vi "RWRPrompt.vi"(0 "Value Present in Detector 2":string) -> (1 "Value to update in Detector 2":string="0000", 2 "Cancel Pressed":bool)   [LabVIEW 2018]
panel:
  in  "Cancel":bool
  in  "Update":bool
  in  "Value to update in Detector":string="0000"
  out "Value Present in Detector":string
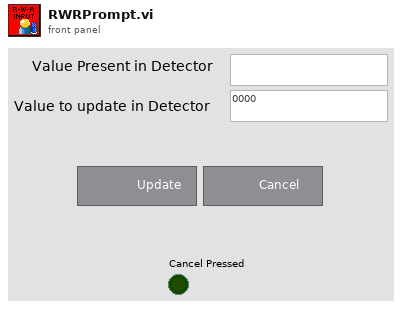
[diagram p1: front panel]
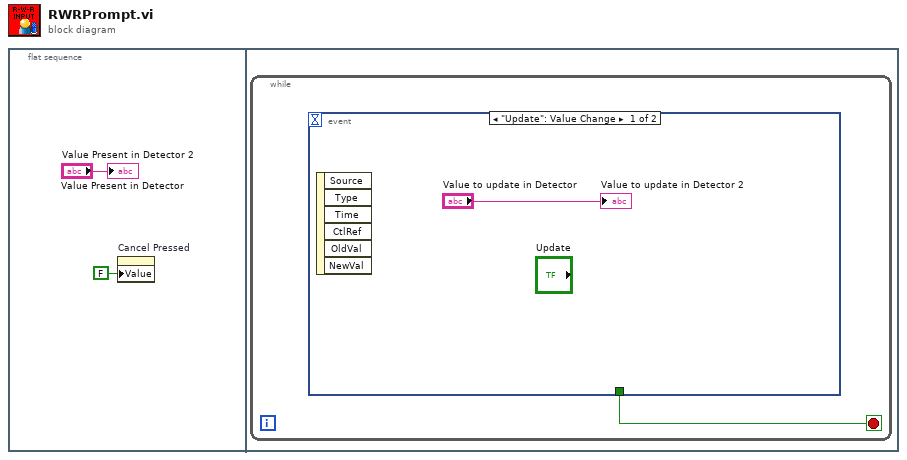
[diagram p0: block diagram]
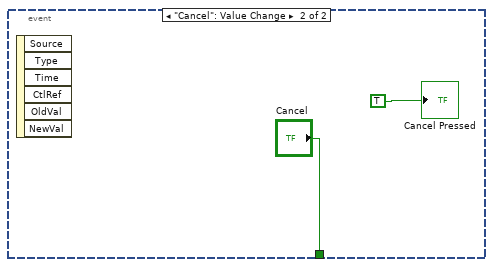
[diagram p2: hidden frame]
diagram:
  n1 = flat-sequence {
    frame #0 {
      n2 = property on="Cancel Pressed" class="Bool (strict)"("Value"=FALSE ("Cancel Pressed")) -> ()  [unwired: 2 in, 2 out]
      "Value Present in Detector" <- "Value Present in Detector 2"
    }
    frame #1 {
      n3 = while {
        stop <- w3 stop-if-true
        n4 = event shown="[0] \"Update\": Value Change" {
          selector: _ -> [_ _]
          dyn-events: _ -> [_ _]
          timeout: _ -> [_ _]
          tunnel: [_ "Cancel"] -> w3
          event "Update": Value Change {
            n5 = event-data() -> ()  [unwired: 1 in, 6 out]
            "Value to update in Detector 2" <- "Value to update in Detector"
          }
          event "Cancel": Value Change {
            n6 = event-data() -> ()  [unwired: 1 in, 6 out]
            "Cancel Pressed" <- TRUE
          }
        }
      }
    }
  }
